vi "Move_Arm_to_Card_Dropoff.vi"(9 "index":i32=19, 10 "error in":errorcluster, 11 "Machine In":refnum<visa-resource-name>) -> (2 "error out":errorcluster, 3 "Machine Out":refnum<visa-resource-name>)   [LabVIEW 2018]
doc: "Example interface for controlling uArm Swift Pro."
panel:
  in  "Write Buffer":string="G90 G0 X1\n"
  out "read buffer":string
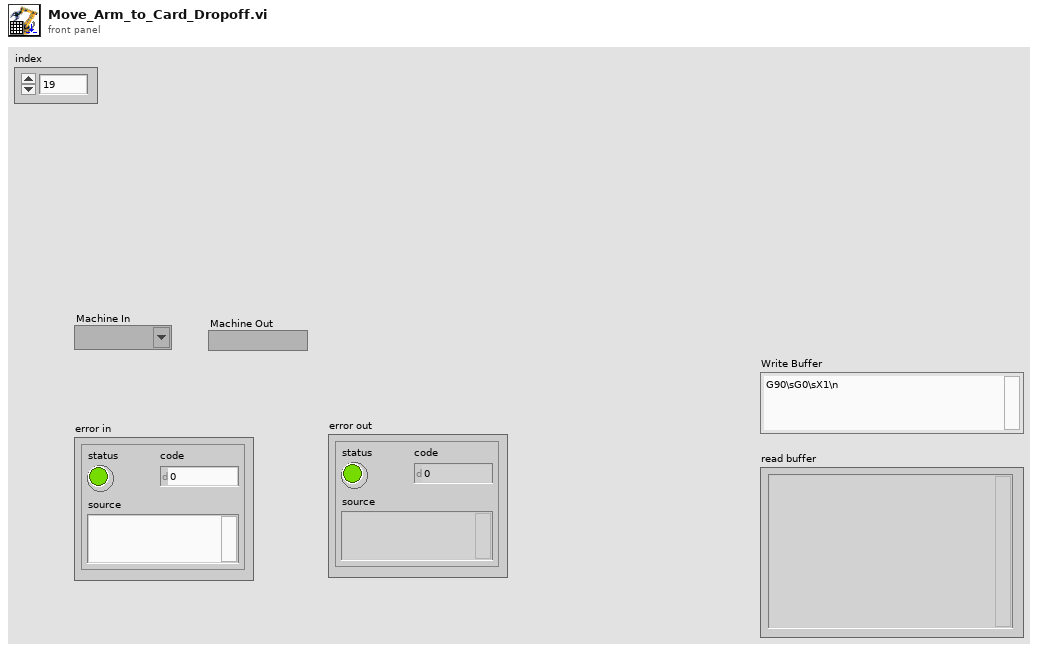
[diagram p1: front panel]
types:
  T1 = cluster{"Numeric Control":dbl, "Numeric Control":dbl}[]
  T2 = cluster{"Numeric Control":dbl, "Numeric Control":dbl}
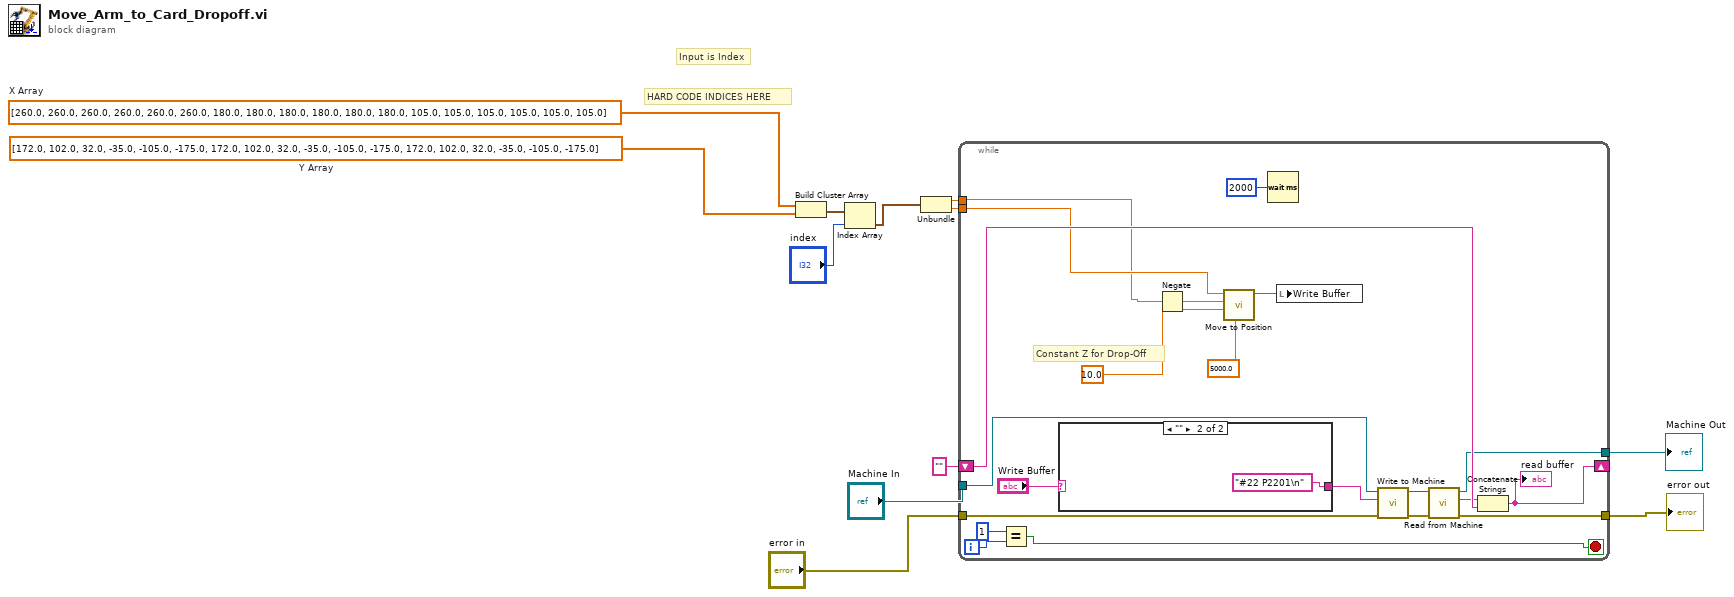
[diagram p0: block diagram]
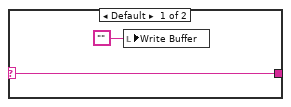
[diagram p2: hidden frame]
diagram:
  w10 = dbl[] [172.0, 102.0, 32.0, -35.0, -105.0, -175.0, 172.0, 102.0, 32.0, -35.0, -105.0, -175.0, 172.0, 102.0, 32.0, -35.0, -105.0, -175.0]  # Y Array
  w11 = dbl[] [260.0, 260.0, 260.0, 260.0, 260.0, 260.0, 180.0, 180.0, 180.0, 180.0, 180.0, 180.0, 105.0, 105.0, 105.0, 105.0, 105.0, 105.0]  # X Array
  # "HARD CODE INDICES HERE"
  # "Input is Index"
  n1 = Build Cluster Array(w11, w10) -> (w9:T1)
  n2 = Index Array(array=w9, index="index") -> (element=w8:T2)
  n3 = Unbundle(w8) -> ("Numeric Control"=w6:dbl, "Numeric Control"=w7:dbl)
  n4 = while {
    tunnel: "Machine In" -> [w31]
    tunnel: "error in" -> [w28]
    shift-right: [w29] -> _
    shift-left: "" -> [w30]
    tunnel: [w27] -> w2
    tunnel: [w23] -> w1
    tunnel: w7 -> [w19]
    tunnel: w6 -> [w18]
    i -> [w16]
    stop <- w14 stop-if-true
    # "Constant Z for Drop-Off"
    n5 = Equal?(x=1, y=w16) -> (x = y?=w14:bool)
    n6 = case shown="\"\"" "Write Buffer" {
      selector: "Write Buffer" -> [w35 _]
      tunnel: [w35 "#22 P2201\n"] -> w32
      frame Default {
        n7 = local write "Write Buffer"("") -> ()
      }
      frame "" {
      }
    }
    n8 = Negate(x=w18) -> (-x=w21:dbl)
    n9 = call "Move to Position.vi"("Speed"=5000.0, "Z-Position"=10.0, "Y-Position"=w21, "X-Position"=w19) -> ("G-Code String"=w22:string)  [unwired: 7 in]
    n10 = Wait (ms)(milliseconds to wait=u32 2000) -> ()  [unwired: 1 out]
    n11 = local write "Write Buffer"(w22) -> ()
    n12 = call "Write to Machine .vi"("error in (no error)"=w28, "G-Code String In"=w32, "Machine In"=w31) -> ("error out"=w25:errorcluster, "Machine Out"=w24:refnum<visa-resource-name>)  [unwired: 7 in]
    n13 = call "Read from Machine.vi"("error in (no error)"=w25, "Machine In"=w24) -> ("error out"=w23:errorcluster, "read buffer"=w26:string, "Machine Out"=w27:refnum<visa-resource-name>)  [unwired: 7 in]
    n14 = Concatenate Strings(w26, w30) -> (w29:string)
    "read buffer" <- w29
  }
  "Machine Out" <- w2
  "error out" <- w1
